vi "Connect Camera A615.vi"() -> ()   [LabVIEW 2015]
uses:
  <vilib>/userdefined/High Color/IMAQdx.ctl
  <vilib>/vision/driver/NI_Vision_Acquisition_Software.lvlib
  <resource>/objmgr/imaqdx.rc
panel:
  out "Temperature":dbl(slide) scale=0.0..40.0
  out "Image":T1(plugin-control)
  in  "Stop":bool
  in  "Session In":T2
  # "Please select the camera you want to access the thermal image"
  # "Note: The Image control needs to be set to 16-bit display. This is done by with the following steps\n            1) Right click on the Image display and select 16-Bit Display Mapping to bring up Set 16 Bit Display Mapping window\n            2) Un-tick \"Apply mapping only when Configured bit depth is 0\" in the Set 16 Bit Display Mapping window\n            3) Set the Conversion Method to Full Dynamic if not already selected"
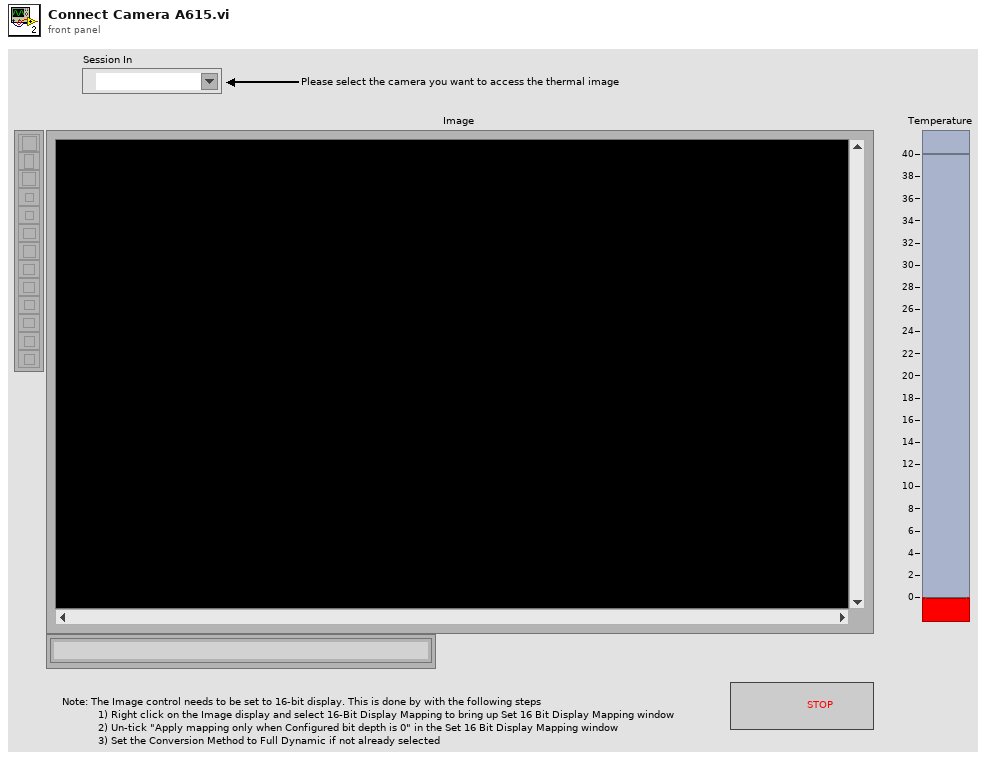
[diagram p1: front panel]
types:
  T1 = typedef "IMAQ Image.ctl" = refnum<image>
  T2 = typedef "IMAQdx.ctl" = refnum<k21>
  T3 = typedef "Image Type" = u32
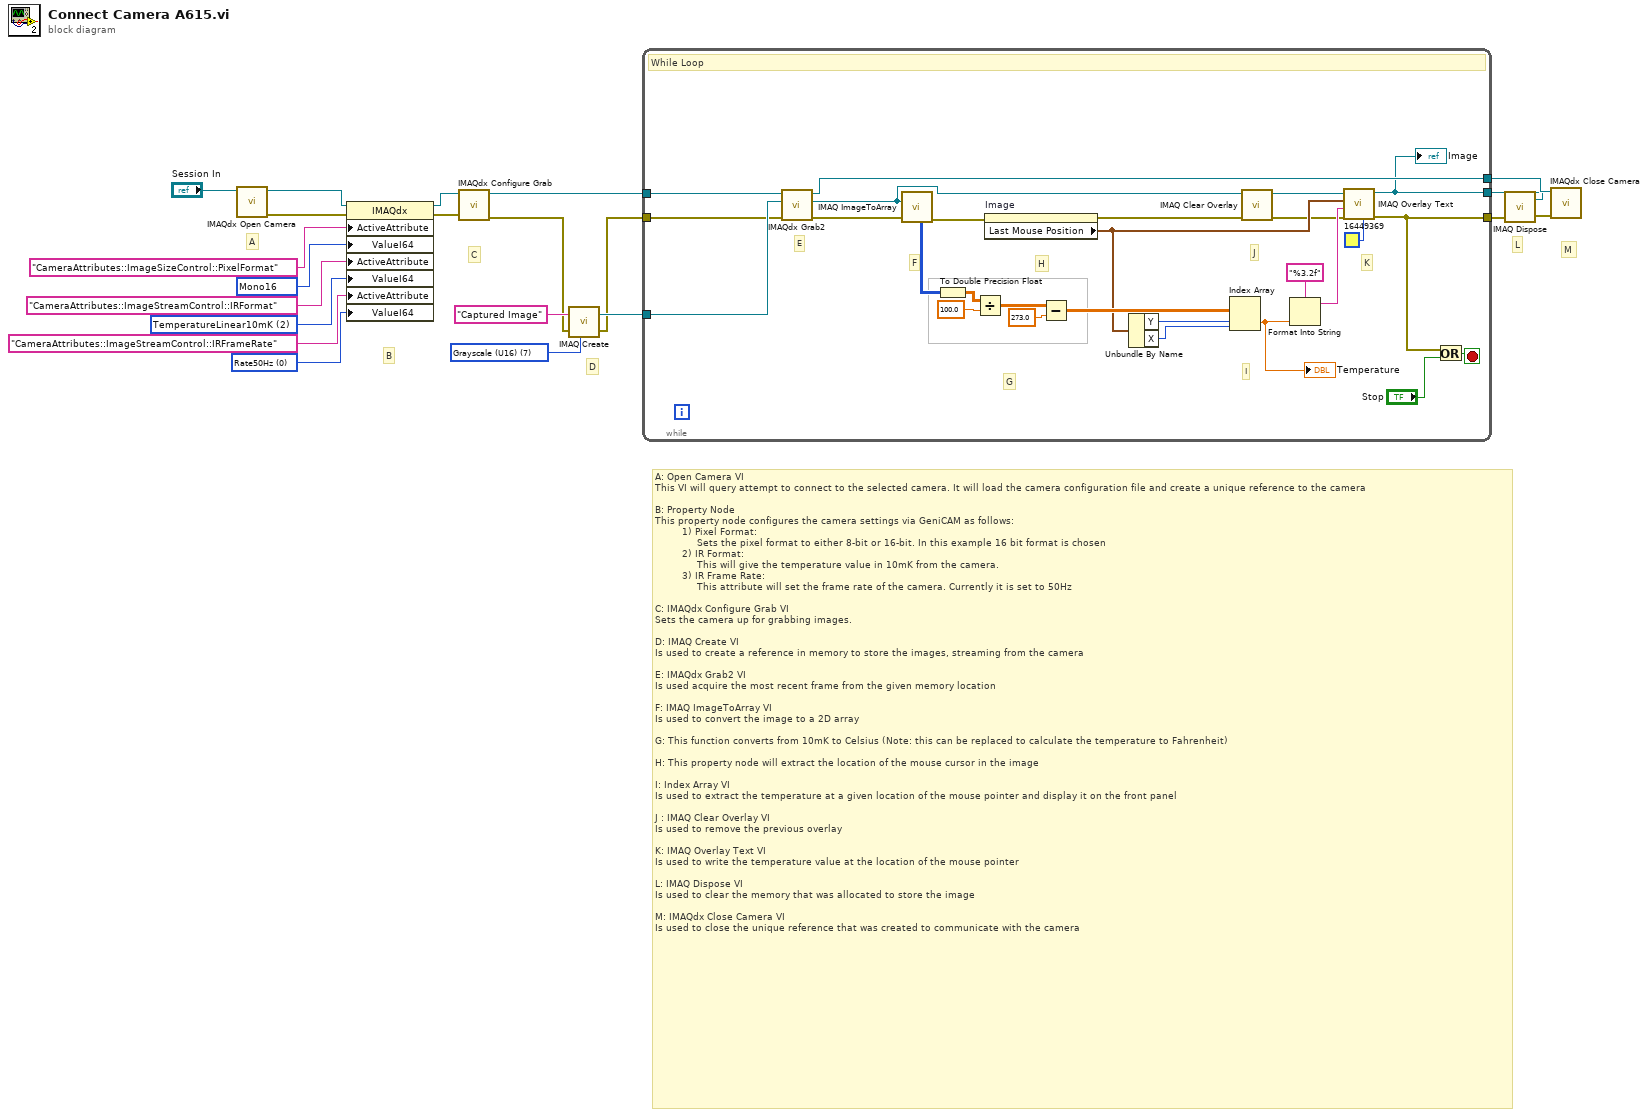
[diagram p0: block diagram]
diagram:
  w7 = i64 0 items=["Rate50Hz"=0, "Rate25Hz"=1, "Rate12Hz"=2, "Rate6Hz"=4, "Rate3Hz"=5] ("IRFrameRate")
  w8 = i64 2 items=["Radiometric", "TemperatureLinear100mK", "TemperatureLinear10mK"] ("IRFormat")
  w11 = i64 17825799 items=["Mono 8"=17301505, "Mono8Signed"=17301506, "Mono10"=17825795, "Mono10Packed"=17563652, "Mono12"=17825797, "Mono12Packed"=17563654, "Mono16"=17825799] ("Ring")
  w16 = T3 7 items=["Grayscale (U8)", "Grayscale (I16)", "Grayscale (SGL)", "Complex (CSG)", "RGB (U32)", "HSL (U32)", "RGB (U64)", "Grayscale (U16)"] ("Image Type")
  # "M"
  # "L"
  # "A: Open Camera VI\nThis VI will query attempt to connect to the selected camera. It will load the camera configuration file and create a unique reference to the camera\n\nB: Property Node\nThis property node configures the camera settings via GeniCAM as follows:\n         1) Pixel Format:\n              Sets the pixel format to either 8-bit or 16-bit. In this example 16 bit format is chosen\n         2) IR Format:\n              This will give the temperature value in 10mK from the camera.\n         3) IR Frame Rate:\n              This attribute will set the frame rate of the camera. Currently it is set to 50Hz\n\nC: IMAQdx Configure Grab VI\nSets the camera up for grabbing images.\n\nD: IMAQ Create VI\nIs used to create a reference in memory to store the images, streaming from the camera\n\nE: IMAQdx Grab2 VI\nIs used acquire the most recent frame from the given memory location\n\nF: IMAQ ImageToArray VI\nIs used to convert the image to a 2D array\n\nG: This function converts from 10mK to Celsius (Note: this can be replaced to calculate the temperature to Fahrenheit)\n\nH: This property node will extract the location of the mouse cursor in the image\n\nI: Index Array VI\nIs used to extract the temperature at a given location of the mouse pointer and display it on the front panel\n\nJ : IMAQ Clear Overlay VI\nIs used to remove the previous overlay\n\nK: IMAQ Overlay Text VI\nIs used to write the temperature value at the location of the mouse pointer\n\nL: IMAQ Dispose VI\nIs used to clear the memory that was allocated to store the image\n\nM: IMAQdx Close Camera VI\nIs used to close the unique reference that was created to communicate with the camera"
  # "D"
  # "C"
  # "B"
  # "A"
  n1 = call <vilib>:"IMAQdx Open Camera.vi"("Session In"="Session In") -> ("error out"=w20:errorcluster, "Session Out"=w13:T2)  [unwired: 9 in]
  n2 = property class="IMAQdx"(reference=w13, error in=w20, "ActiveAttribute"="CameraAttributes::ImageSizeControl::PixelFormat", "ValueI64"=w11, "ActiveAttribute"="CameraAttributes::ImageStreamControl::IRFormat", "ValueI64"=w8, "ActiveAttribute"="CameraAttributes::ImageStreamControl::IRFrameRate", "ValueI64"=w7) -> (reference out=w19:T2, error out=w6:errorcluster)
  n3 = call <vilib>:"IMAQdx Configure Grab.vi"("error in"=w6, "Session In"=w19) -> ("error out"=w5:errorcluster, "Session Out"=w18:T2)  [unwired: 8 in]
  n4 = call "IMAQ Create"("Image Name"="Captured Image", "Image Type"=w16, "error in (no error)"=w5) -> ("New Image"=w15:T1, "error out"=w4:errorcluster)  [unwired: 2 in]
  n5 = while {
    tunnel: w4 -> [w42]
    tunnel: w18 -> [w48]
    tunnel: w15 -> [w44]
    tunnel: [w47] -> w14
    tunnel: [w26] -> w2
    tunnel: [w22] -> w3
    stop <- w46 stop-if-true
    # "K"
    # "J"
    # "I"
    # "H"
    # "G"
    # "F"
    # "E"
    # "While Loop"
    n6 = call <vilib>:"IMAQdx Grab2.vi"("error in"=w42, "Image In"=w44, "Session In"=w48) -> ("error out"=w43:errorcluster, "Image Out"=w29:T1, "Session Out"=w47:T2)  [unwired: 5 in, 1 out]
    n7 = call "IMAQ ImageToArray"("error in (no error)"=w43, "Image"=w29) -> ("Image Pixels (U16)"=w41:u16[][], "error out"=w39:errorcluster)  [unwired: 2 in, 3 out]
    n8 = To Double Precision Float(number=w41) -> (double precision float=w38:dbl[][])
    n9 = Divide(x=w38, y=100.0) -> (x/y=w35:dbl[][])
    n10 = property on="Image" class="ImageControl"(error in=w39) -> (error out=w27:errorcluster, "Last Mouse Position"=w30:cluster{"X":i32, "Y":i32})  [unwired: 1 in, 1 out]
    n11 = Subtract(x=w35, y=273.0) -> (x-y=w40:dbl[][])
    n12 = Unbundle By Name(w30) -> ("Y"=w23:i32, "X"=w24:i32)
    n13 = Index Array(array=w40, index (row)=w23, index (col)=w24) -> (element=w34:dbl)
    "Temperature" <- w34
    n14 = call "IMAQ Clear Overlay"("error in (no error)"=w27, "Image"=w29) -> ("error out"=w25:errorcluster, "Image Out"=w28:T1)  [unwired: 8 in]
    n15 = Format Into String(format string="%3.2f", w34) -> (resulting string=w32:string)  [unwired: 2 in, 1 out]
    n16 = call "IMAQ Overlay Text"("BG Color (Transparent)"=u32 16449369, "error in (no error)"=w25, "String"=w32, "Origin"=w30, "Image"=w28) -> ("error out"=w26:errorcluster, "Image Out"=w22:T1)  [unwired: 5 in]
    "Image" <- w22
    n17 = Or(x=w26, y="Stop") -> (x .or. y?=w46:bool)
  }
  n18 = call "IMAQ Dispose"("Image"=w3, "error in (no error)"=w2) -> ("error out"=w1:errorcluster)  [unwired: 4 in]
  n19 = call <vilib>:"IMAQdx Close Camera.vi"("error in"=w1, "Session In"=w14) -> ()  [unwired: 9 in, 1 out]
